vi "vim instance string array to var array.vi"(11 "Array in":string[](array[string])) -> (3 "Array out":variant[](array[variant]))   [LabVIEW 2025, in "LUnit Extensions Tests.lvclass"]
uses:
  LUnit Extensions Tests.lvclass
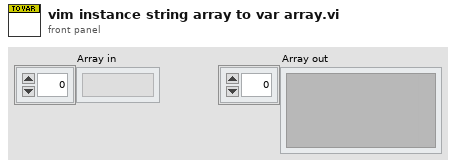
[diagram p1: front panel]
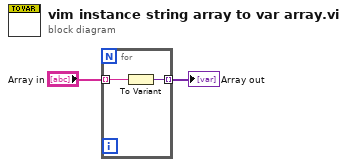
[diagram p0: block diagram]
diagram:
  n1 = for {
    tunnel: "Array in" -> [w4] mode=indexing
    tunnel: [w3] -> w2 mode=indexing
    n2 = To Variant(anything=w4) -> (Variant=w3:variant)
  }
  "Array out" <- w2
